vi "Init.vi"(8 "error in (no error)":errorcluster, 11 "DAQmx Base CFG in":refnum<class "DAQmx Base CFG.lvclass">) -> (0 "error out":errorcluster, 3 "DAQmx Base CFG out":refnum<class "DAQmx Base CFG.lvclass">)   [LabVIEW 2023, in "DAQmx Base CFG.lvclass"]
uses:
  DAQmx Base CFG.lvclass
  DAQmx Base CFG.lvclass/DAQmx Base CFG.ctl
  <vilib>/Utility/error.llb/Error Cluster From Error Code.vi
  <vilib>/ErrorRing/Error Ring.xnode
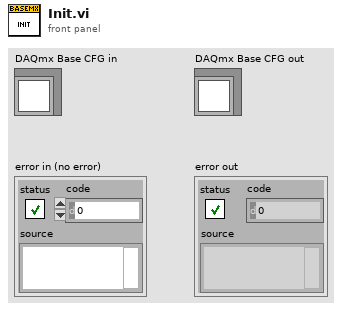
[diagram p1: front panel]
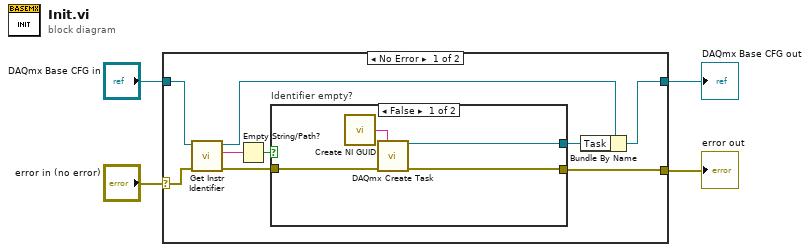
[diagram p0: block diagram]
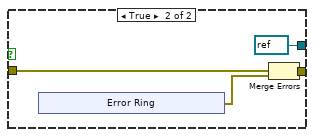
[diagram p2: hidden frame]
diagram:
  n1 = case shown="No Error" "error in (no error)" {
    selector: "error in (no error)" -> [w13 w27]
    tunnel: "DAQmx Base CFG in" -> [w12 w28]
    tunnel: [w6 w28] -> w2
    tunnel: [w8 w27] -> w1
    frame No Error {
      n2 = call-dynamic "Get Instr Identifier.vi"("error in (no error)"=w13, "Configuration Base in"=w12) -> ("error out"=w9:errorcluster, "Instr Identifier"=w11:string, "Configuration Base out"=w7:refnum<class "DAQmx Base CFG.lvclass">)  [unwired: 7 in]
      n3 = Empty String/Path?(string/path=w11) -> (empty?=w10:bool)
      n4 = case "Identifier empty?" shown="False" w10 {
        tunnel: w9 -> [w17 w21]
        tunnel: [w16 w20] -> w8
        tunnel: [w14 refnum<k21> refnum ("task out")] -> w5
        frame False {
          n5 = call <vilib>:"Create NI GUID.vi"() -> ("NI GUID"=w15:string)
          n6 = call <vilib>:"DAQmx Create Task.vi"("new task name"=w15, "error in"=w17) -> ("task out"=w14:refnum<k21>, "error out"=w16:errorcluster)  [unwired: 12 in]
        }
        frame True {
          n7 = xnode "Error Ring"() -> ("error out"=w19:errorcluster)
          n8 = Merge Errors(w21, w19) -> (w20:errorcluster)
        }
      }
      n9 = Bundle By Name(cluster=w7, "Task"=w5) -> (w6:refnum<class "DAQmx Base CFG.lvclass">)
    }
    frame Error {
    }
  }
  "error out" <- w1
  "DAQmx Base CFG out" <- w2
